vi "ex1b.vi"() -> ()   [LabVIEW 2022 SP3]
panel:
  out "Array":i32[][](array[numeric])
  in  "dimension size":i32
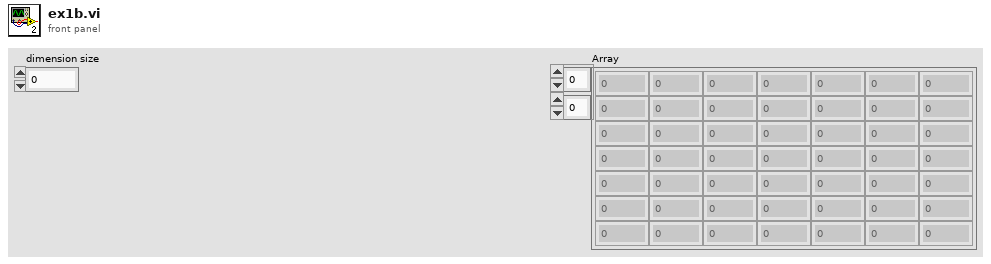
[diagram p1: front panel]
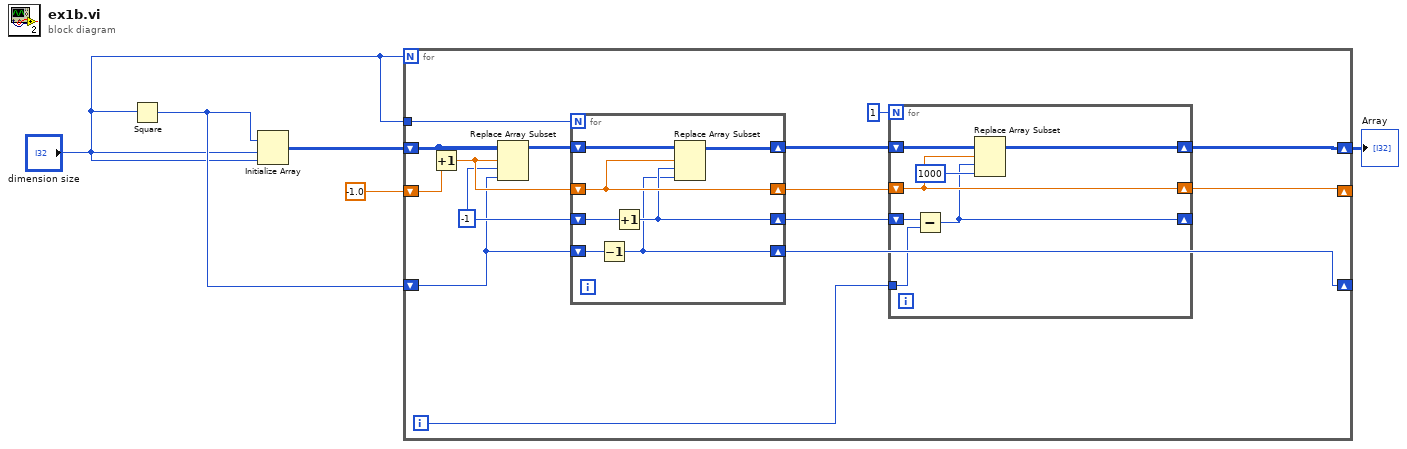
[diagram p0: block diagram]
diagram:
  n1 = Square(x="dimension size") -> (x^2=w4:i32)
  n2 = Initialize Array(w4, "dimension size", "dimension size") -> (w5:i32[][])
  n3 = for {
    N: "dimension size" -> [_]
    shift-right: [w11] -> w1
    shift-left: w5 -> [w16]
    shift-right: [w9] -> _
    shift-left: w4 -> [w14]
    shift-right: [w10] -> _
    shift-left: -1.0 -> [w19]
    tunnel: "dimension size" -> [w15]
    i -> [w6]
    w17 = -1
    n4 = Increment(x=w19) -> (x+1=w18:dbl)
    n5 = Replace Array Subset(array=w16, new element=w14, index (row)=w18, index (col)=w17) -> ()  [unwired: 1 out]
    n6 = for {
      N: w15 -> [_]
      shift-right: [w29] -> w12
      shift-left: w18 -> [w29]
      shift-right: [w28] -> w7
      shift-left: w17 -> [w33]
      shift-right: [w30] -> w13
      shift-left: w16 -> [w32]
      shift-right: [w27] -> w9
      shift-left: w14 -> [w31]
      n7 = Decrement(x=w31) -> (x-1=w27:i32)
      n8 = Increment(x=w33) -> (x+1=w28:i32)
      n9 = Replace Array Subset(array=w32, new element=w27, index (row)=w29, index (col)=w28) -> (w30:i32[][])
    }
    n10 = for {
      N: 1 -> [_]
      shift-right: [w24] -> w11
      shift-left: w13 -> [w26]
      shift-right: [w23] -> w10
      shift-left: w12 -> [w23]
      shift-right: [w21] -> _
      shift-left: w7 -> [w20]
      tunnel: w6 -> [w22]
      n11 = Subtract(x=w20, y=w22) -> (x-y=w21:i32)
      n12 = Replace Array Subset(array=w26, new element=1000 ("new element/subarray"), index (row)=w23, index (col)=w21) -> (w24:i32[][])
    }
  }
  "Array" <- w1
